vi "coerce.vi"(7 "dimension":T1, 8 "error in (no error)":errorcluster, 10 "coordinates in":dbl[unit][](array[numeric]), 11 "Box in":refnum<class "Box.lvclass">) -> (0 "error out":errorcluster, 1 "coerced?":bool[](array[boolean]), 2 "coordinates out":dbl[unit][](array[numeric]), 3 "Box out":refnum<class "Box.lvclass">, 4 "in range?":bool[](array[boolean]))   [LabVIEW 2010, in "Box.lvclass"]
uses:
  Box.lvclass
  enumerations/x_y_z_enumeration.ctl
  Box.lvclass/Box.ctl
  SpaceVector/SpaceVector/SpaceVector.lvclass
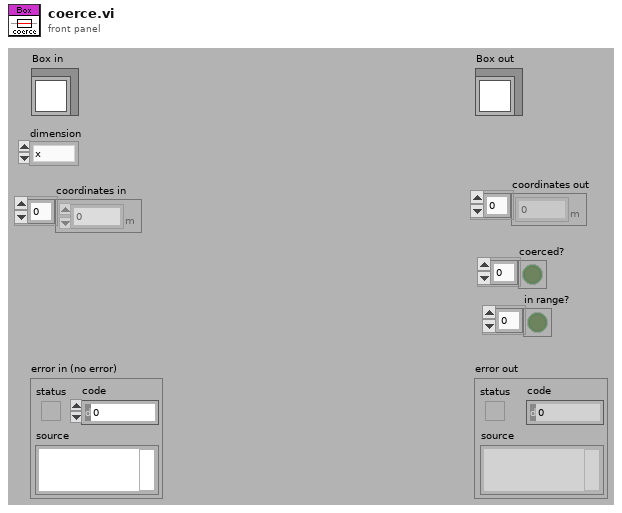
[diagram p1: front panel]
types:
  T1 = typedef "x_y_z_enumeration.ctl" = enum16{"x", "y", "z"}
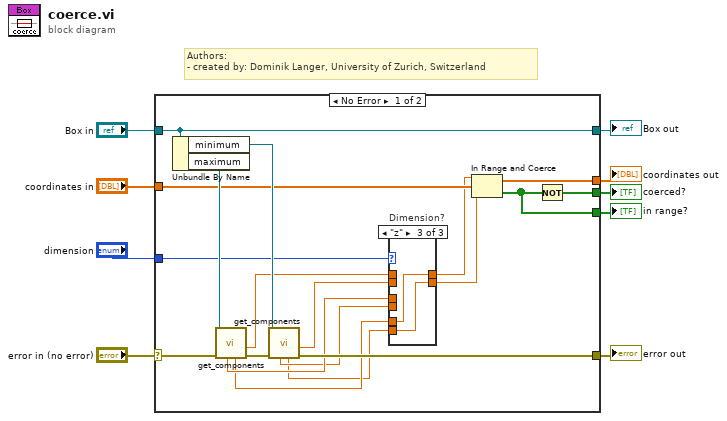
[diagram p0: block diagram]
diagram:
  # "Authors: \n- created by: Dominik Langer, University of Zurich, Switzerland"
  n1 = case shown="No Error" "error in (no error)" {
    selector: "error in (no error)" -> [w24 w36]
    tunnel: [w23 w36] -> w8
    tunnel: [w28 w35] -> w6
    tunnel: "Box in" -> [w28 w35]
    tunnel: "dimension" -> [w21 _]
    tunnel: "coordinates in" -> [w22 _]
    tunnel: [w12 _] -> w4
    tunnel: [w11 _] -> w3
    tunnel: [w10 _] -> w2
    frame No Error {
      n2 = Unbundle By Name(w28) -> ("minimum"=w26:refnum<class "SpaceVector.lvclass">, "maximum"=w27:refnum<class "SpaceVector.lvclass">)
      n3 = call "get_components.vi"("error in (no error)"=w24, "SpaceVector in"=w27) -> ("error out"=w25:errorcluster, "x"=w20:dbl[unit], "z"=w16:dbl[unit], "y"=w18:dbl[unit])  [unwired: 6 out]
      n4 = call "get_components.vi"("error in (no error)"=w25, "SpaceVector in"=w26) -> ("error out"=w23:errorcluster, "x"=w19:dbl[unit], "z"=w15:dbl[unit], "y"=w17:dbl[unit])  [unwired: 6 out]
      n5 = case "Dimension?" shown="\"z\"" w21 {
        tunnel: w20 -> [w30 _ _]
        tunnel: w19 -> [w29 _ _]
        tunnel: w18 -> [_ w32 _]
        tunnel: w17 -> [_ w31 _]
        tunnel: w16 -> [_ _ w34]
        tunnel: w15 -> [_ _ w33]
        tunnel: [w30 w32 w34] -> w14
        tunnel: [w29 w31 w33] -> w13
        frame "x", Default {
        }
        frame "y" {
        }
        frame "z" {
        }
      }
      n6 = In Range and Coerce(upper limit=w14, x=w22, lower limit=w13) -> (coerced(x)=w12:dbl[unit][], In Range?=w10:bool[])
      n7 = Not(x=w10) -> (.not. x?=w11:bool[])
    }
    frame Error {
    }
  }
  "error out" <- w8
  "Box out" <- w6
  "coordinates out" <- w4
  "coerced?" <- w3
  "in range?" <- w2
